vi "Create balloon 队列.vi"() -> (3 "队列输出":refnum<queue>)   [LabVIEW 2016, in "斯坦道总磷总氮.lvlib"]
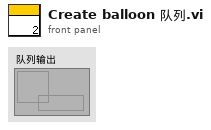
[diagram p1: front panel]
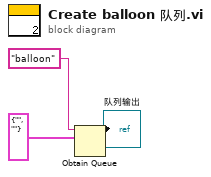
[diagram p0: block diagram]
diagram:
  n1 = Obtain Queue(name (unnamed)="balloon" ("名称（未命名）"), element data type=cluster{"Title":string, "Body":string} {"Title"="", "Body"=""}) -> (queue out=→"队列输出":refnum<queue>)  [unwired: 3 in, 2 out]
